vi "GetSerialNumber.vi"(8 "error in":errorcluster, 11 "VISA resource name":refnum<visa-resource-name>) -> (0 "error out":errorcluster, 2 "Chamber serial number":string, 3 "VISA resource name out":refnum<visa-resource-name>)   [LabVIEW 2023, in "Thermotron 8800.lvlib"]
doc: "SERL\nCommand name: Send chamber serial number\nCommand type: System status\nDescription: This query command asks the 8800 for the chamber’s serial number.\nSyntax: SERL?\nData type: Integer\nQuery example: SERL?\n8800 response: 42679 (The chamber’s serial number is 42679)"
uses:
  Thermotron 8800.lvlib
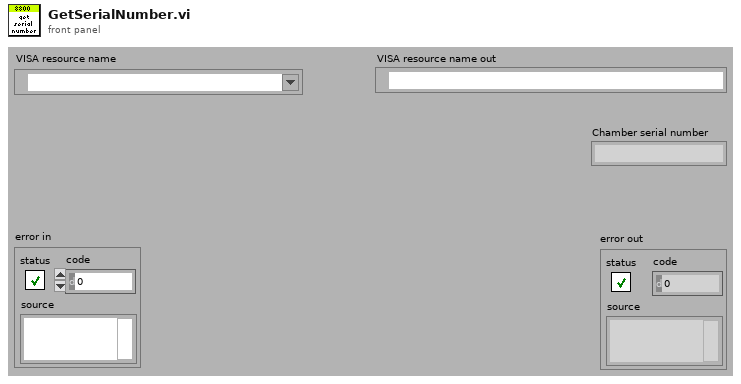
[diagram p1: front panel]
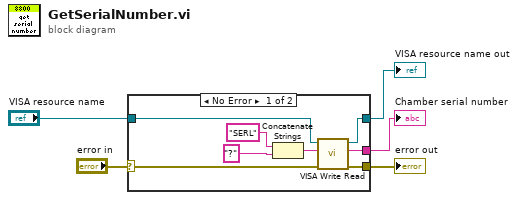
[diagram p0: block diagram]
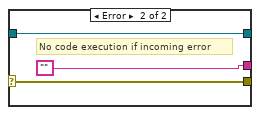
[diagram p2: hidden frame]
diagram:
  n1 = case shown="No Error" "error in" {
    selector: "error in" -> [w11 w16]
    tunnel: [w10 w16] -> w4
    tunnel: "VISA resource name" -> [w9 w14]
    tunnel: [w8 w14] -> w2
    tunnel: [w7 ""] -> w1
    frame No Error {
      n2 = Concatenate Strings("SERL" ("8800 Command"), "?" ("8800 Command")) -> (w13:string)
      n3 = call "VISA Write Read.vi"("error in (no error)"=w11, "8800 Command"=w13, "VISA Refnum in"=w9) -> ("error out"=w10:errorcluster, "read buffer"=w7:string, "VISA Refnum out"=w8:refnum<visa-resource-name>)  [unwired: 6 in]
    }
    frame Error {
      # "No code execution if incoming error"
    }
  }
  "error out" <- w4
  "VISA resource name out" <- w2
  "Chamber serial number" <- w1
